vi "Lookup Model Serial.vi"(8 "error in (no error)":errorcluster, 9 "Serial":string, 10 "Model":string, 11 "SensorList in":refnum<class "SensorList.lvclass">) -> (0 "error out":errorcluster, 2 "Sensor":refnum<class "Sensor.lvclass">, 3 "SensorList out":refnum<class "SensorList.lvclass">)   [LabVIEW 2020, in "VolatusConfig.lvlib" / "SensorList.lvclass"]
uses:
  SensorList.lvclass
  C:/dev/lv20CE/relink/lv-volatus/VolatusConfig/VolatusConfigElement/VolatusConfigElement.lvclass
  Sensor/Sensor.lvclass
  VolatusConfigElement/VolatusConfigElement.lvclass/VolatusConfigElement.ctl
  VolatusConfigElement/VolatusConfigElement.lvclass
  lv-cdm/CDM-Config/Config Element/Config Element.lvclass
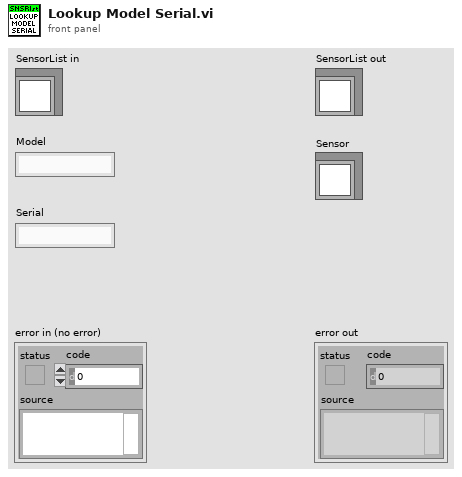
[diagram p1: front panel]
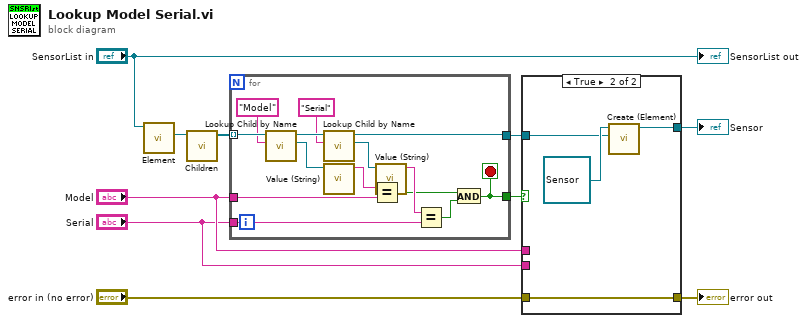
[diagram p0: block diagram]
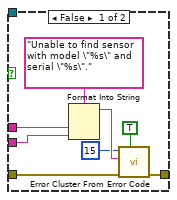
[diagram p2: hidden frame]
diagram:
  n1 = call "Element.vi"("VolatusConfigElement in"="SensorList in") -> ("Element"=w9:refnum<class "Config Element.lvclass">)  [unwired: 9 in, 1 out]
  n2 = call "Children.vi"("Config Element in"=w9) -> ("Elements"=w8:refnum<class "Config Element.lvclass">[])  [unwired: 9 in, 1 out]
  n3 = for {
    tunnel: w8 -> [w24] mode=indexing
    tunnel: "Model" -> [w17]
    tunnel: "Serial" -> [w16]
    tunnel: [w12] -> w7
    tunnel: [w11] -> w6
    stop <- w11 stop-if-true
    n4 = call "Lookup Child by Name.vi"("Name"="Model", "Config Element in"=w24) -> ("Child"=w20:refnum<class "Config Element.lvclass">, "Config Element out"=w22:refnum<class "Config Element.lvclass">)  [unwired: 6 in, 2 out]
    n5 = call "Lookup Child by Name.vi"("Name"="Serial", "Config Element in"=w22) -> ("Child"=w19:refnum<class "Config Element.lvclass">, "Config Element out"=w12:refnum<class "Config Element.lvclass">)  [unwired: 6 in, 2 out]
    n6 = call "Value (String).vi"("Config Element in"=w20) -> ("String Value"=w18:string)  [unwired: 9 in, 1 out]
    n7 = Equal?(x=w18, y=w17) -> (x = y?=w14:bool)
    n8 = call "Value (String).vi"("Config Element in"=w19) -> ("String Value"=w15:string)  [unwired: 9 in, 1 out]
    n9 = Equal?(x=w15, y=w16) -> (x = y?=w13:bool)
    n10 = And(x=w14, y=w13) -> (x .and. y?=w11:bool)
  }
  n11 = case shown="True" w6 {
    tunnel: w7 -> [_ w34]
    tunnel: "error in (no error)" -> [w32 w36]
    tunnel: "Model" -> [w29 _]
    tunnel: "Serial" -> [w28 _]
    tunnel: [w31 w36] -> w2
    tunnel: [_ w33] -> w1
    frame False {
      n12 = Format Into String(format string="Unable to find sensor with model \"%s\" and serial \"%s\".", w29, w28) -> (resulting string=w26:string)  [unwired: 2 in, 1 out]
      n13 = call <vilib>:"Error Cluster From Error Code.vi"("show call chain? (False)"=TRUE, "error in (no error)"=w32, "error message (\"\")"=w26, "error code (0)"=15) -> ("error out"=w31:errorcluster)  [unwired: 5 in]
    }
    frame True {
      n14 = call "Create (Element).vi"("Element"=w34, "VolatusConfigElement in"=refnum<class "Sensor.lvclass"> refnum ("VolatusConfig.lvlib:Sensor")) -> ("VolatusConfigElement out"=w33:refnum<class "Sensor.lvclass">)  [unwired: 8 in, 1 out]
    }
  }
  "error out" <- w2
  "Sensor" <- w1
  "SensorList out" <- "SensorList in"
